vi "Cubehelix.vi"(11 "Fraction (0 to 1)":dbl) -> (3 "RGB Hex Value":u32 format="%06x")   [LabVIEW 2015]
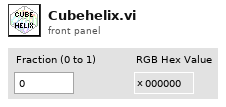
[diagram p1: front panel]
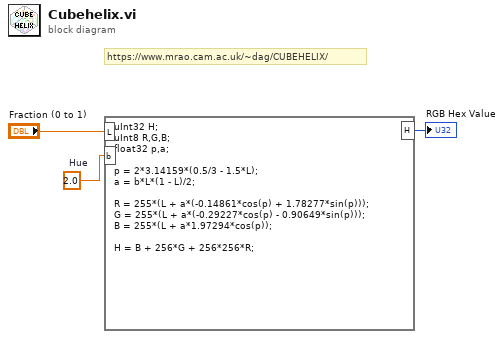
[diagram p0: block diagram]
diagram:
  w1 = 2.0  # Hue
  # "https://www.mrao.cam.ac.uk/~dag/CUBEHELIX/"
  n1 = formula code="uInt32 H;\nuInt8 R,G,B;\nfloat32 p,a;\n\np = 2*3.14159*(0.5/3 - 1.5*L);\na = b*L*(1 - L)/2;\n\nR = 255*(L + a*(-0.14861*cos(p) + 1.78277*sin(p)));\nG = 255*(L + a*(-0.29227*cos(p) - 0.90649*sin(p)));\nB = 255*(L + a*1.97294*cos(p));\n\nH = B + 256*G + 256*256*R;"("L"="Fraction (0 to 1)", "b"=w1) -> ("H"=→"RGB Hex Value":u32)
